vi "main-all-channels.vi"() -> ()   [LabVIEW 2024]
uses:
  controls/thermocouple-input-cluster.ctl
  controls/analog-input-cluster.ctl
  controls/analog-output-cluster.ctl
  controls/digitial-input-cluster.ctl
  controls/digital-output-cluster.ctl
  controls/adam-module-select-tab.ctl
  controls/adam-5000-serial-settings.ctl
  controls/adam-5000-cmd-response.ctl
  controls/state-enum.ctl
  controls/adam-5000-all-chassis-data.ctl
  controls/adam-5000-all-module-datas.ctl
  controls/adam-5000-chassis-cmd-ack.ctl
  controls/adam-5000-chassis-module-types.ctl
  controls/adam-5000-DO-user-input.ctl
  controls/adam-5000-AO-user-input.ctl
panel:
  out "cmd-response:7":T1
  out "status-indicator:7":cluster{"Sampling":bool, "Ack":bool}
  in  "Slot 7: Module Type":T2(ring)=enum."empty"
  out "slot: 7":T3
  in  "7:Digital Outputs":T4
  out "7:Digital Inputs":T5
  in  "7:Analog Outputs":T6
  out "7:Analog Inputs":T7
  out "7:Thermocouple Inputs (degC)":T8
  out "cmd-response:6":T1
  out "status-indicator:6":cluster{"Sampling":bool, "Ack":bool}
  in  "Slot 6: Module Type":T2(ring)=enum."empty"
  out "slot: 6":T3
  in  "6:Digital Outputs":T4
  out "6:Digital Inputs":T5
  in  "6:Analog Outputs":T6
  out "6:Analog Inputs":T7
  out "6:Thermocouple Inputs (degC)":T8
  out "cmd-response:5":T1
  out "status-indicator:5":cluster{"Sampling":bool, "Ack":bool}
  in  "Slot 5: Module Type":T2(ring)=enum."Analog Output"
  out "slot: 5":T3
  in  "5:Digital Outputs":T4
  out "5:Digital Inputs":T5
  in  "5:Analog Outputs":T6
  out "5:Analog Inputs":T7
  out "5:Thermocouple Inputs (degC)":T8
  out "cmd-response:4":T1
  out "status-indicator:4":cluster{"Sampling":bool, "Ack":bool}
  in  "Slot 4: Module Type":T2(ring)=enum."Power Relay"
  out "slot: 4":T3
  in  "4:Digital Outputs":T4
  out "4:Digital Inputs":T5
  in  "4:Analog Outputs":T6
  out "4:Analog Inputs":T7
  out "4:Thermocouple Inputs (degC)":T8
  out "cmd-response:3":T1
  out "status-indicator:3":cluster{"Sampling":bool, "Ack":bool}
  in  "Slot 3: Module Type":T2(ring)=enum."Thermocouple"
  out "slot: 3":T3
  in  "3:Digital Outputs":T4
  out "3:Digital Inputs":T5
  in  "3:Analog Outputs":T6
  out "3:Analog Inputs":T7
  out "3:Thermocouple Inputs (degC)":T8
  out "cmd-response:2":T1
  out "status-indicator:2":cluster{"Sampling":bool, "Ack":bool}
  in  "Slot 2: Module Type":T2(ring)=enum."Analog Input"
  out "slot: 2":T3
  in  "2:Digital Outputs":T4
  out "2:Digital Inputs":T5
  in  "2:Analog Outputs":T6
  out "2:Analog Inputs":T7
  out "2:Thermocouple Inputs (degC)":T8
  out "cmd-response:1":T1
  out "status-indicator:1":cluster{"Sampling":bool, "Ack":bool}
  in  "Slot 1: Module Type":T2(ring)=enum."Thermocouple"
  out "slot: 1":T3
  in  "1:Digital Outputs":T4
  out "1:Digital Inputs":T5
  in  "1:Analog Outputs":T6
  out "1:Analog Inputs":T7
  out "1:Thermocouple Inputs (degC)":T8
  out "cmd-response:0":T1
  out "status-indicator:0":cluster{"Sampling":bool, "Ack":bool}
  in  "Slot 0: Module Type":T2(ring)=enum."Analog Input"
  out "slot: 0":T3
  in  "0:Digital Outputs":T4
  out "0:Digital Inputs":T5
  in  "0:Analog Outputs:":T6
  out "0:Analog Inputs":T7
  out "0:Thermocouple Inputs (degC)":T8
  out "Current Slot":i32
  in  "Chassis Settings":T9={"VISA resource name"="COM8", "baud rate (19200)"=19200, "Chassis ID"=1}
  out "Loop Time (mS)":u32
  out "Loop Counter":i32
  out "Write Success":bool
  out "error IO":errorcluster
  out "error":errorcluster
  in  "exit":bool
  # "ADAM 5000 Controller"
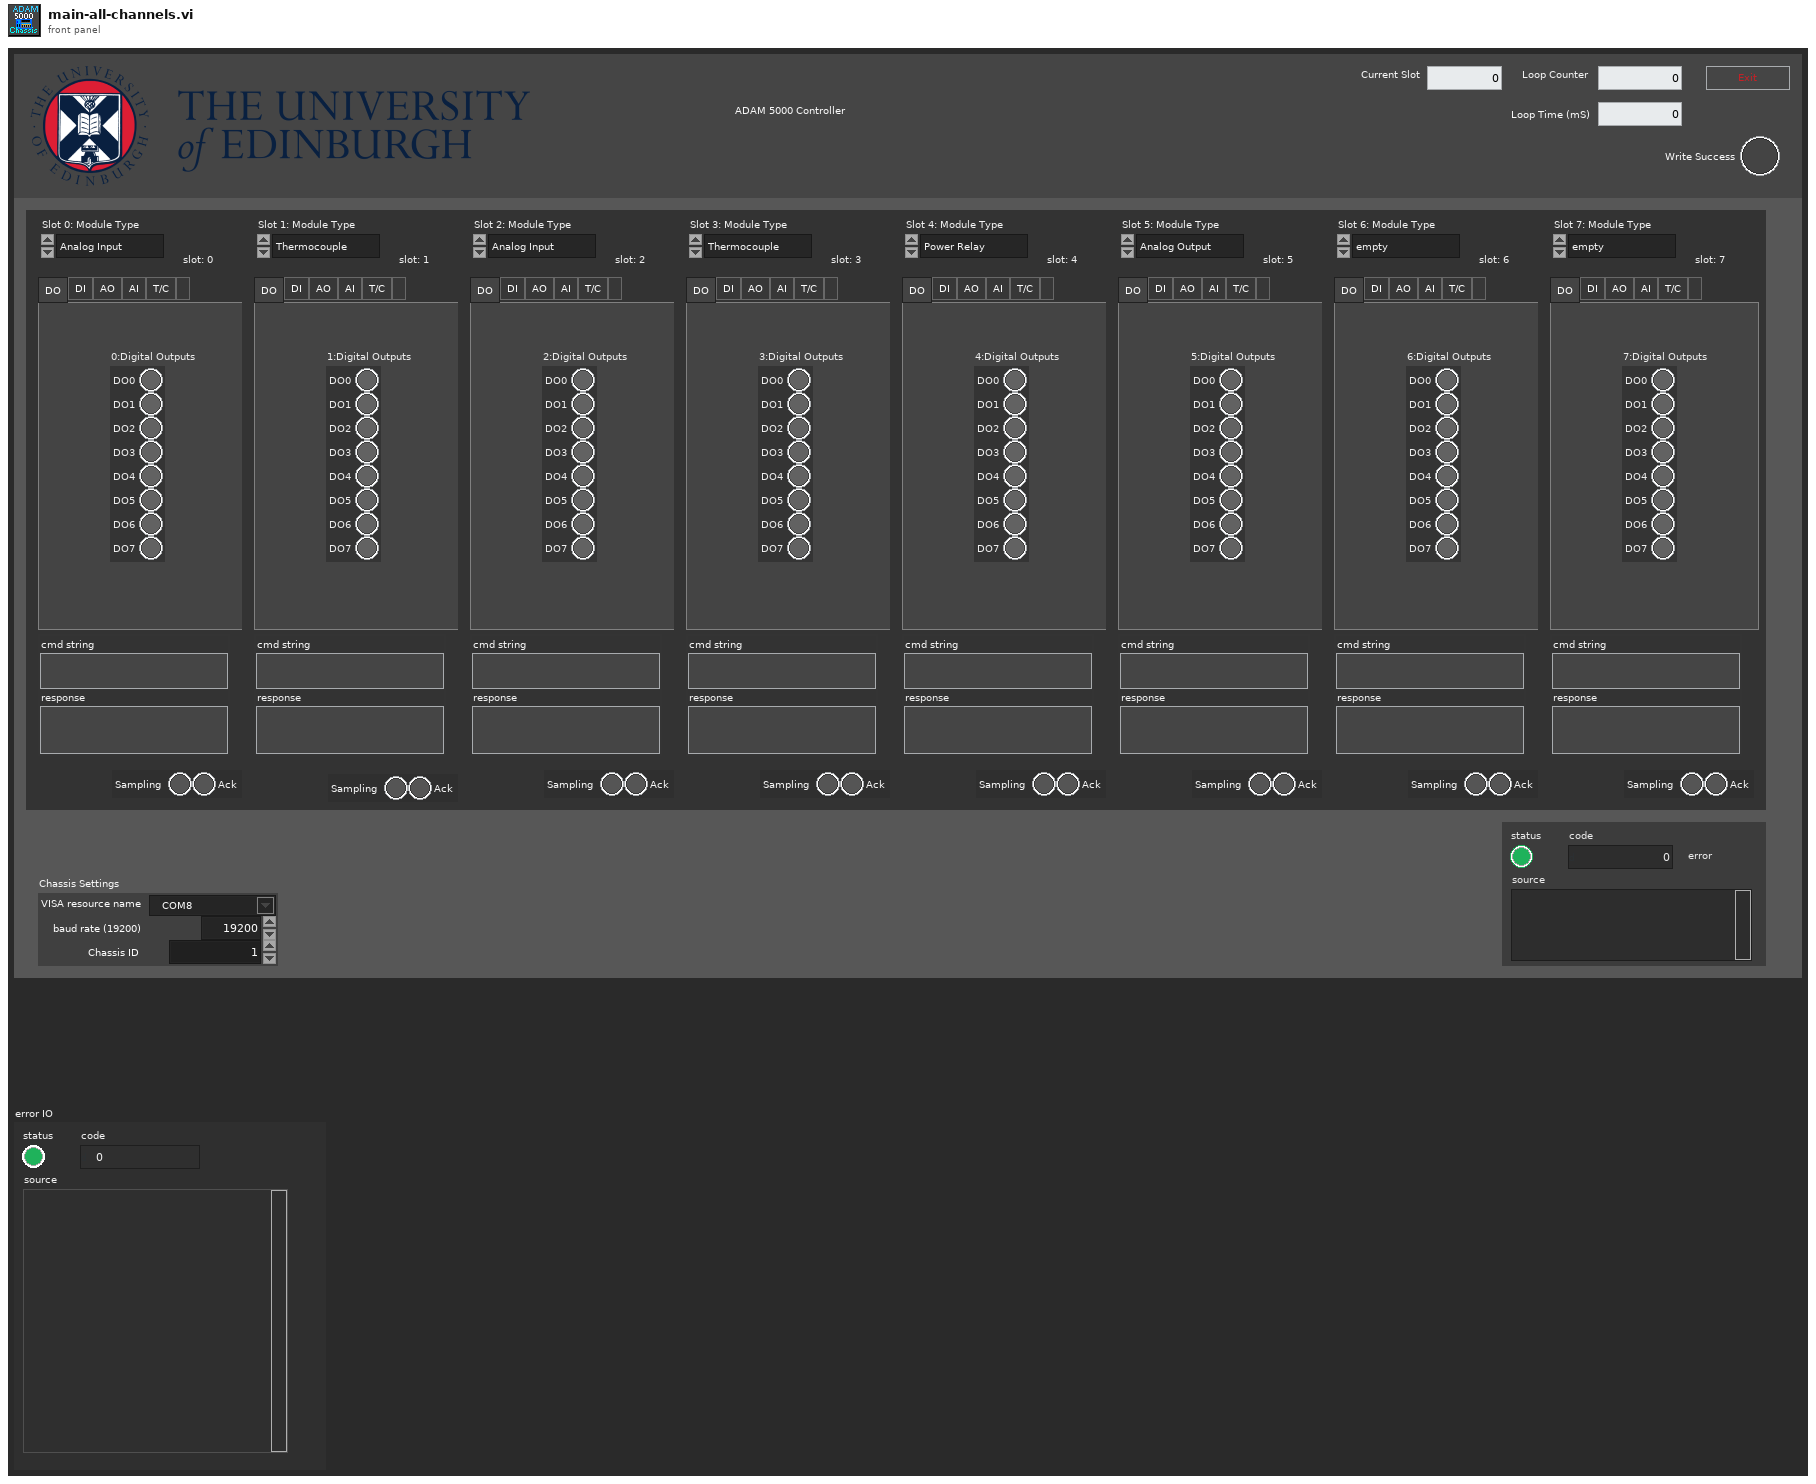
[diagram p1: front panel]
types:
  T1 = typedef "adam-5000-cmd-response.ctl" = cluster{"cmd string":string, "response":string}
  T2 = enum16{"Digital Output", "Digital Input", "Analog Output", "Analog Input", "Thermocouple", "Power Relay", "empty"}
  T3 = typedef "adam-module-select-tab.ctl" = enum32{"DO", "DI", "AO", "AI", "T/C", ""}
  T4 = typedef "digital-output-cluster.ctl" = cluster{"DO0":bool, "DO1":bool, "DO2":bool, "DO3":bool, "DO4":bool, "DO5":bool, "DO6":bool, "DO7":bool}
  T5 = typedef "digitial-input-cluster.ctl" = cluster{"DI0":bool, "DI1":bool, "DI2":bool, "DI3":bool, "DI4":bool, "DI5":bool, "DI6":bool, "DI7":bool}
  T6 = typedef "analog-output-cluster.ctl" = cluster{"AO0":dbl, "AO1":dbl, "AO2":dbl, "AO3":dbl}
  T7 = typedef "analog-input-cluster.ctl" = cluster{"AI0":dbl, "AI1":dbl, "AI2":dbl, "AI3":dbl, "AI4":dbl, "AI5":dbl, "AI6":dbl, "AI7":dbl}
  T8 = typedef "thermocouple-input-cluster.ctl" = cluster{"TC0":dbl, "TC1":dbl, "TC2":dbl, "TC3":dbl, "TC4":dbl, "TC5":dbl, "TC6":dbl}
  T9 = typedef "adam-5000-serial-settings.ctl" = cluster{"VISA resource name":refnum<visa-resource-name>, "baud rate (19200)":u32, "Chassis ID":u8}
  T10 = typedef "adam-5000-chassis-cmd-ack.ctl" = cluster{"cmd-response:0":T1, "cmd-response:1":T1, "cmd-response:2":T1, "cmd-response:3":T1, "cmd-response:4":T1, "cmd-response:5":T1, "cmd-response:6":T1, "cmd-response:7":T1}
  T11 = typedef "adam-5000-all-chassis-data.ctl" = cluster{"slot:0":T12, "slot:1":T12, "slot:2":T12, "slot:3":T12, "slot:4":T12, "slot:5":T12, "slot:6":T12, "slot:7":T12}
  T12 = typedef "adam-5000-all-module-datas.ctl" = cluster{"Digital Outputs":T4, "Digital Inputs":T5, "Analog Outputs":T6, "Analog Inputs":T7, "Thermocouple Inputs (degC)":T8}
  T13 = typedef "state-enum.ctl" = enum16{"init", "wait", "manual", "start", "run", "reset", "stop", "exit"}
  T14 = typedef "adam-5000-AO-user-input.ctl" = cluster{"0:Analog Outputs":T6, "1:Analog Outputs":T6, "2:Analog Outputs":T6, "3:Analog Outputs":T6, "4:Analog Outputs":T6, "5:Analog Outputs":T6, "6:Analog Outputs":T6, "7:Analog Outputs":T6}
  T15 = typedef "adam-5000-DO-user-input.ctl" = cluster{"0:Digital Outputs":T4, "1:Digital Outputs":T4, "2:Digital Outputs":T4, "3:Digital Outputs":T4, "4:Digital Outputs":T4, "5:Digital Outputs":T4, "6:Digital Outputs":T4, "7:Digital Outputs":T4}
  T16 = typedef "adam-5000-chassis-module-types.ctl" = cluster{"Slot 0: Module Type":enum16{"Digital Output", "Digital Input", "Analog Output", "Analog Input", "Thermocouple", "Power Relay", "empty"}, "Slot 1: Module Type":enum16{"Digital Output", "Digital Input", "Analog Output", "Analog Input", "Thermocouple", "Power Relay", "empty"}, "Slot 2: Module Type":enum16{"Digital Output", "Digital Input", "Analog Output", "Analog Input", "Thermocouple", "Power Relay", "empty"}, "Slot 3: Module Type":enum16{"Digital Output", "Digital Input", "Analog Output", "Analog Input", "Thermocouple", "Power Relay", "empty"}, "Slot 4: Module Type":enum16{"Digital Output", "Digital Input", "Analog Output", "Analog Input", "Thermocouple", "Power Relay", "empty"}, "Slot 5: Module Type":enum16{"Digital Output", "Digital Input", "Analog Output", "Analog Input", "Thermocouple", "Power Relay", "empty"}, "Slot 6: Module Type":enum16{"Digital Output", "Digital Input", "Analog Output", "Analog Input", "Thermocouple", "Power Relay", "empty"}, "Slot 7: Module Type":enum16{"Digital Output", "Digital Input", "Analog Output", "Analog Input", "Thermocouple", "Power Relay", "empty"}}
  T17 = cluster{"status-indicator:0":refnum<vi>, "status-indicator:1":refnum<vi>, "status-indicator:2":refnum<vi>, "status-indicator:3":refnum<vi>, "status-indicator:4":refnum<vi>, "status-indicator:5":refnum<vi>, "status-indicator:6":refnum<vi>, "status-indicator:7":refnum<vi>}
  T18 = enum16{"Digital Output", "Digital Input", "Analog Output", "Analog Input", "Thermocouple", "Power Relay", "empty"}[]
  T19 = cluster{"[0]":T3, "[1]":T3, "[2]":T3, "[3]":T3, "[4]":T3, "[5]":T3, "[6]":T3, "[7]":T3, "[8]":T3}
  T20 = cluster{"[0]":T12, "[1]":T12, "[2]":T12, "[3]":T12, "[4]":T12, "[5]":T12, "[6]":T12, "[7]":T12, "[8]":T12}
  T21 = cluster{"[0]":T1, "[1]":T1, "[2]":T1, "[3]":T1, "[4]":T1, "[5]":T1, "[6]":T1, "[7]":T1, "[8]":T1}
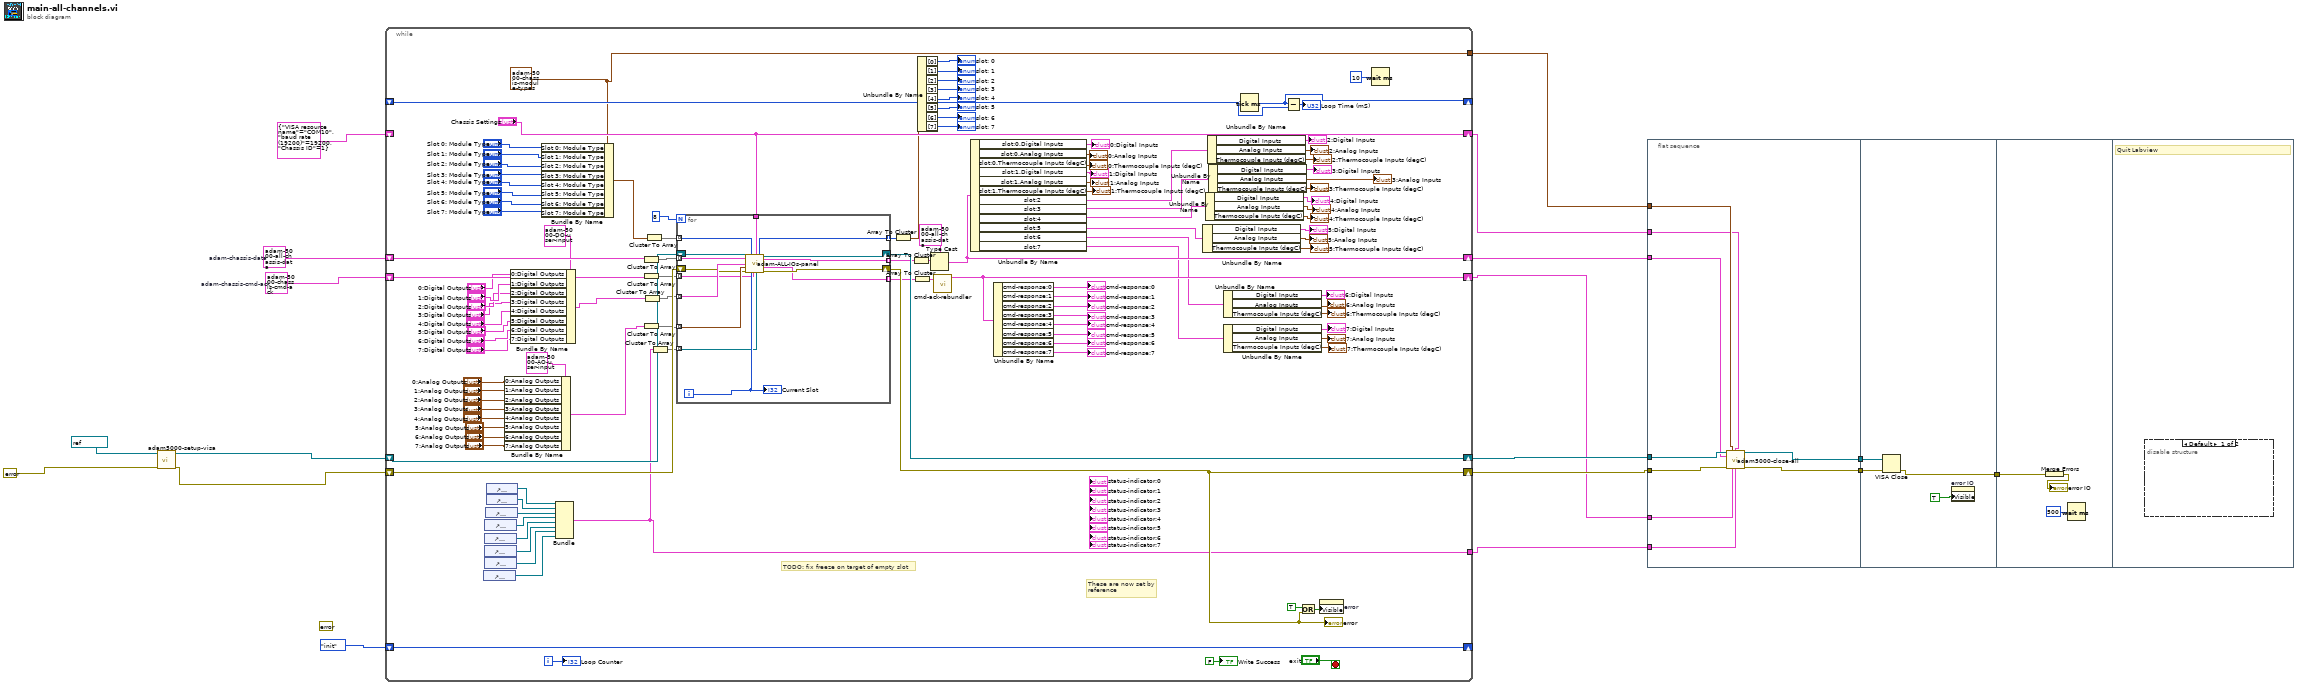
[diagram p0: block diagram]
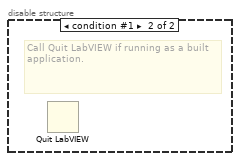
[diagram p2: hidden frame]
diagram:
  w10 = T10 {"cmd-response:0"={"cmd string"="", "response"=""}, "cmd-response:1"={"cmd string"="", "response"=""}, "cmd-response:2"={"cmd string"="", "response"=""}, "cmd-response:3"={"cmd string"="", "response"=""}, "cmd-response:4"={"cmd string"="", "response"=""}, "cmd-response:5"={"cmd string"="", "response"=""}, "cmd-response:6"={"cmd string"="", "response"=""}, "cmd-response:7"={"cmd string"="", "response"=""}}  # adam-chassis-cmd-ack
  w11 = T11 {"slot:0"={"Digital Outputs"={"DO0"=FALSE, "DO1"=FALSE, "DO2"=FALSE, "DO3"=FALSE, "DO4"=FALSE, "DO5"=FALSE, "DO6"=FALSE, "DO7"=FALSE}, "Digital Inputs"={"DI0"=FALSE, "DI1"=FALSE, "DI2"=FALSE, "DI3"=FALSE, "DI4"=FALSE, "DI5"=FALSE, "DI6"=FALSE, "DI7"=FALSE}, "Analog Outputs"={"AO0"=0.0, "AO1"=0.0, "AO2"=0.0, "AO3"=0.0}, "Analog Inputs"={"AI0"=0.0, "AI1"=0.0, "AI2"=0.0, "AI3"=0.0, "AI4"=0.0, "AI5"=0.0, "AI6"=0.0, "AI7"=0.0}, "Thermocouple Inputs (degC)"={"TC0"=0.0, "TC1"=0.0, "TC2"=0.0, "TC3"=0.0, "TC4"=0.0, "TC5"=0.0, "TC6"=0.0}}, "slot:1"={"Digital Outputs"={"DO0"=FALSE, "DO1"=FALSE, "DO2"=FALSE, "DO3"=FALSE, "DO4"=FALSE, "DO5"=FALSE, "DO6"=FALSE, "DO7"=FALSE}, "Digital Inputs"={"DI0"=FALSE, "DI1"=FALSE, "DI2"=FALSE, "DI3"=FALSE, "DI4"=FALSE, "DI5"=FALSE, "DI6"=FALSE, "DI7"=FALSE}, "Analog Outputs"={"AO0"=0.0, "AO1"=0.0, "AO2"=0.0, "AO3"=0.0}, "Analog Inputs"={"AI0"=0.0, "AI1"=0.0, "AI2"=0.0, "AI3"=0.0, "AI4"=0.0, "AI5"=0.0, "AI6"=0.0, "AI7"=0.0}, "Thermocouple Inputs (degC)"={"TC0"=0.0, "TC1"=0.0, "TC2"=0.0, "TC3"=0.0, "TC4"=0.0, "TC5"=0.0, "TC6"=0.0}}, "slot:2"={"Digital Outputs"={"DO0"=FALSE, "DO1"=FALSE, "DO2"=FALSE, "DO3"=FALSE, "DO4"=FALSE, "DO5"=FALSE, "DO6"=FALSE, "DO7"=FALSE}, "Digital Inputs"={"DI0"=FALSE, "DI1"=FALSE, "DI2"=FALSE, "DI3"=FALSE, "DI4"=FALSE, "DI5"=FALSE, "DI6"=FALSE, "DI7"=FALSE}, "Analog Outputs"={"AO0"=0.0, "AO1"=0.0, "AO2"=0.0, "AO3"=0.0}, "Analog Inputs"={"AI0"=0.0, "AI1"=0.0, "AI2"=0.0, "AI3"=0.0, "AI4"=0.0, "AI5"=0.0, "AI6"=0.0, "AI7"=0.0}, "Thermocouple Inputs (degC)"={"TC0"=0.0, "TC1"=0.0, "TC2"=0.0, "TC3"=0.0, "TC4"=0.0, "TC5"=0.0, "TC6"=0.0}}, "slot:3"={"Digital Outputs"={"DO0"=FALSE, "DO1"=FALSE, "DO2"=FALSE, "DO3"=FALSE, "DO4"=FALSE, "DO5"=FALSE, "DO6"=FALSE, "DO7"=FALSE}, "Digital Inputs"={"DI0"=FALSE, "DI1"=FALSE, "DI2"=FALSE, "DI3"=FALSE, "DI4"=FALSE, "DI5"=FALSE, "DI6"=FALSE, "DI7"=FALSE}, "Analog Outputs"={"AO0"=0.0, "AO1"=0.0, "AO2"=0.0, "AO3"=0.0}, "Analog Inputs"={"AI0"=0.0, "AI1"=0.0, "AI2"=0.0, "AI3"=0.0, "AI4"=0.0, "AI5"=0.0, "AI6"=0.0, "AI7"=0.0}, "Thermocouple Inputs (degC)"={"TC0"=0.0, "TC1"=0.0, "TC2"=0.0, "TC3"=0.0, "TC4"=0.0, "TC5"=0.0, "TC6"=0.0}}, "slot:4"={"Digital Outputs"={"DO0"=FALSE, "DO1"=FALSE, "DO2"=FALSE, "DO3"=FALSE, "DO4"=FALSE, "DO5"=FALSE, "DO6"=FALSE, "DO7"=FALSE}, "Digital Inputs"={"DI0"=FALSE, "DI1"=FALSE, "DI2"=FALSE, "DI3"=FALSE, "DI4"=FALSE, "DI5"=FALSE, "DI6"=FALSE, "DI7"=FALSE}, "Analog Outputs"={"AO0"=0.0, "AO1"=0.0, "AO2"=0.0, "AO3"=0.0}, "Analog Inputs"={"AI0"=0.0, "AI1"=0.0, "AI2"=0.0, "AI3"=0.0, "AI4"=0.0, "AI5"=0.0, "AI6"=0.0, "AI7"=0.0}, "Thermocouple Inputs (degC)"={"TC0"=0.0, "TC1"=0.0, "TC2"=0.0, "TC3"=0.0, "TC4"=0.0, "TC5"=0.0, "TC6"=0.0}}, "slot:5"={"Digital Outputs"={"DO0"=FALSE, "DO1"=FALSE, "DO2"=FALSE, "DO3"=FALSE, "DO4"=FALSE, "DO5"=FALSE, "DO6"=FALSE, "DO7"=FALSE}, "Digital Inputs"={"DI0"=FALSE, "DI1"=FALSE, "DI2"=FALSE, "DI3"=FALSE, "DI4"=FALSE, "DI5"=FALSE, "DI6"=FALSE, "DI7"=FALSE}, "Analog Outputs"={"AO0"=0.0, "AO1"=0.0, "AO2"=0.0, "AO3"=0.0}, "Analog Inputs"={"AI0"=0.0, "AI1"=0.0, "AI2"=0.0, "AI3"=0.0, "AI4"=0.0, "AI5"=0.0, "AI6"=0.0, "AI7"=0.0}, "Thermocouple Inputs (degC)"={"TC0"=0.0, "TC1"=0.0, "TC2"=0.0, "TC3"=0.0, "TC4"=0.0, "TC5"=0.0, "TC6"=0.0}}, "slot:6"={"Digital Outputs"={"DO0"=FALSE, "DO1"=FALSE, "DO2"=FALSE, "DO3"=FALSE, "DO4"=FALSE, "DO5"=FALSE, "DO6"=FALSE, "DO7"=FALSE}, "Digital Inputs"={"DI0"=FALSE, "DI1"=FALSE, "DI2"=FALSE, "DI3"=FALSE, "DI4"=FALSE, "DI5"=FALSE, "DI6"=FALSE, "DI7"=FALSE}, "Analog Outputs"={"AO0"=0.0, "AO1"=0.0, "AO2"=0.0, "AO3"=0.0}, "Analog Inputs"={"AI0"=0.0, "AI1"=0.0, "AI2"=0.0, "AI3"=0.0, "AI4"=0.0, "AI5"=0.0, "AI6"=0.0, "AI7"=0.0}, "Thermocouple Inputs (degC)"={"TC0"=0.0, "TC1"=0.0, "TC2"=0.0, "TC3"=0.0, "TC4"=0.0, "TC5"=0.0, "TC6"=0.0}}, "slot:7"={"Digital Outputs"={"DO0"=FALSE, "DO1"=FALSE, "DO2"=FALSE, "DO3"=FALSE, "DO4"=FALSE, "DO5"=FALSE, "DO6"=FALSE, "DO7"=FALSE}, "Digital Inputs"={"DI0"=FALSE, "DI1"=FALSE, "DI2"=FALSE, "DI3"=FALSE, "DI4"=FALSE, "DI5"=FALSE, "DI6"=FALSE, "DI7"=FALSE}, "Analog Outputs"={"AO0"=0.0, "AO1"=0.0, "AO2"=0.0, "AO3"=0.0}, "Analog Inputs"={"AI0"=0.0, "AI1"=0.0, "AI2"=0.0, "AI3"=0.0, "AI4"=0.0, "AI5"=0.0, "AI6"=0.0, "AI7"=0.0}, "Thermocouple Inputs (degC)"={"TC0"=0.0, "TC1"=0.0, "TC2"=0.0, "TC3"=0.0, "TC4"=0.0, "TC5"=0.0, "TC6"=0.0}}}  # adam-chassis-data
  (unwired) errorcluster {"status"=FALSE, "code"=0, "source"=""} ("error")
  n1 = call "adam5000-setup-visa.vi"("error in"=errorcluster {"status"=FALSE, "code"=0, "source"=""}, "VISA Refnum in"=refnum<visa-resource-name> "COM8") -> ("error out"=w8:errorcluster, "VISA Refnum out"=w7:refnum<visa-resource-name>)  [unwired: 8 in]
  n2 = while {
    shift-right: [w128] -> _
    shift-left: state-enum."init" ("state-enum") -> [w128]
    shift-right: [w104] -> w17
    shift-left: w8 -> [w116]
    shift-right: [w131] -> _
    shift-left: _ -> [w133]
    shift-right: ["Chassis Settings"] -> w2
    shift-left: T9 {"VISA resource name"="COM10", "baud rate (19200)"=19200, "Chassis ID"=1} ("Chassis Settings") -> [_]
    shift-right: [w115] -> w12
    shift-left: w7 -> [w117]
    shift-right: [w105] -> w5
    shift-left: w11 -> [w114]
    shift-right: [w90] -> w4
    shift-left: w10 -> [w112]
    tunnel: [w20] -> w3
    tunnel: [w19] -> w1
    i -> [w134]
    stop <- "exit" stop-if-true
    w20 = T16 {"Slot 0: Module Type"=enum."Digital Output", "Slot 1: Module Type"=enum."Digital Output", "Slot 2: Module Type"=enum."Digital Output", "Slot 3: Module Type"=enum."Digital Output", "Slot 4: Module Type"=enum."Digital Output", "Slot 5: Module Type"=enum."Digital Output", "Slot 6: Module Type"=enum."Digital Output", "Slot 7: Module Type"=enum."Digital Output"} ("cluster")
    # "TODO: fix freeze on target of empty slot"
    # "These are now set by\nreference"
    n3 = control-ref of="status-indicator:7"() -> (w50:refnum<vi>)
    n4 = control-ref of="status-indicator:4"() -> (w53:refnum<vi>)
    n5 = control-ref of="status-indicator:5"() -> (w52:refnum<vi>)
    n6 = control-ref of="status-indicator:3"() -> (w54:refnum<vi>)
    n7 = control-ref of="status-indicator:6"() -> (w51:refnum<vi>)
    n8 = control-ref of="status-indicator:2"() -> (w84:refnum<vi>)
    n9 = control-ref of="status-indicator:0"() -> (w101:refnum<vi>)
    n10 = control-ref of="status-indicator:1"() -> (w100:refnum<vi>)
    n11 = Bundle By Name(cluster=T14 {"0:Analog Outputs"={"AO0"=0.0, "AO1"=0.0, "AO2"=0.0, "AO3"=0.0}, "1:Analog Outputs"={"AO0"=0.0, "AO1"=0.0, "AO2"=0.0, "AO3"=0.0}, "2:Analog Outputs"={"AO0"=0.0, "AO1"=0.0, "AO2"=0.0, "AO3"=0.0}, "3:Analog Outputs"={"AO0"=0.0, "AO1"=0.0, "AO2"=0.0, "AO3"=0.0}, "4:Analog Outputs"={"AO0"=0.0, "AO1"=0.0, "AO2"=0.0, "AO3"=0.0}, "5:Analog Outputs"={"AO0"=0.0, "AO1"=0.0, "AO2"=0.0, "AO3"=0.0}, "6:Analog Outputs"={"AO0"=0.0, "AO1"=0.0, "AO2"=0.0, "AO3"=0.0}, "7:Analog Outputs"={"AO0"=0.0, "AO1"=0.0, "AO2"=0.0, "AO3"=0.0}}, "0:Analog Outputs"="0:Analog Outputs:", "1:Analog Outputs"="1:Analog Outputs", "2:Analog Outputs"="2:Analog Outputs", "3:Analog Outputs"="3:Analog Outputs", "4:Analog Outputs"="4:Analog Outputs", "5:Analog Outputs"="5:Analog Outputs", "6:Analog Outputs"="6:Analog Outputs", "7:Analog Outputs"="7:Analog Outputs") -> (w29:T14)
    n12 = Bundle By Name(cluster=T15 {"0:Digital Outputs"={"DO0"=FALSE, "DO1"=FALSE, "DO2"=FALSE, "DO3"=FALSE, "DO4"=FALSE, "DO5"=FALSE, "DO6"=FALSE, "DO7"=FALSE}, "1:Digital Outputs"={"DO0"=FALSE, "DO1"=FALSE, "DO2"=FALSE, "DO3"=FALSE, "DO4"=FALSE, "DO5"=FALSE, "DO6"=FALSE, "DO7"=FALSE}, "2:Digital Outputs"={"DO0"=FALSE, "DO1"=FALSE, "DO2"=FALSE, "DO3"=FALSE, "DO4"=FALSE, "DO5"=FALSE, "DO6"=FALSE, "DO7"=FALSE}, "3:Digital Outputs"={"DO0"=FALSE, "DO1"=FALSE, "DO2"=FALSE, "DO3"=FALSE, "DO4"=FALSE, "DO5"=FALSE, "DO6"=FALSE, "DO7"=FALSE}, "4:Digital Outputs"={"DO0"=FALSE, "DO1"=FALSE, "DO2"=FALSE, "DO3"=FALSE, "DO4"=FALSE, "DO5"=FALSE, "DO6"=FALSE, "DO7"=FALSE}, "5:Digital Outputs"={"DO0"=FALSE, "DO1"=FALSE, "DO2"=FALSE, "DO3"=FALSE, "DO4"=FALSE, "DO5"=FALSE, "DO6"=FALSE, "DO7"=FALSE}, "6:Digital Outputs"={"DO0"=FALSE, "DO1"=FALSE, "DO2"=FALSE, "DO3"=FALSE, "DO4"=FALSE, "DO5"=FALSE, "DO6"=FALSE, "DO7"=FALSE}, "7:Digital Outputs"={"DO0"=FALSE, "DO1"=FALSE, "DO2"=FALSE, "DO3"=FALSE, "DO4"=FALSE, "DO5"=FALSE, "DO6"=FALSE, "DO7"=FALSE}}, "0:Digital Outputs"="0:Digital Outputs", "1:Digital Outputs"="1:Digital Outputs", "2:Digital Outputs"="2:Digital Outputs", "3:Digital Outputs"="3:Digital Outputs", "4:Digital Outputs"="4:Digital Outputs", "5:Digital Outputs"="5:Digital Outputs", "6:Digital Outputs"="6:Digital Outputs", "7:Digital Outputs"="7:Digital Outputs") -> (w39:T15)
    n13 = Bundle By Name(cluster=w20, "Slot 0: Module Type"="Slot 0: Module Type", "Slot 1: Module Type"="Slot 1: Module Type", "Slot 2: Module Type"="Slot 2: Module Type", "Slot 3: Module Type"="Slot 3: Module Type", "Slot 4: Module Type"="Slot 4: Module Type", "Slot 5: Module Type"="Slot 5: Module Type", "Slot 6: Module Type"="Slot 6: Module Type", "Slot 7: Module Type"="Slot 7: Module Type") -> (w41:T16)
    n14 = Bundle("status-indicator:0"=w101, "status-indicator:1"=w100, "status-indicator:2"=w84, "status-indicator:3"=w54, "status-indicator:4"=w53, "status-indicator:5"=w52, "status-indicator:6"=w51, "status-indicator:7"=w50) -> (w19:T17)  [unwired: 1 in]
    n15 = Cluster To Array(cluster=w112) -> (array=w111:T1[])
    n16 = Cluster To Array(cluster=w114) -> (array=w113:T12[])
    n17 = Cluster To Array(cluster=w29) -> (array=w109:T6[])
    n18 = Cluster To Array(cluster=w39) -> (array=w110:T4[])
    n19 = Cluster To Array(cluster=w41) -> (array=w103:T18)
    n20 = Cluster To Array(cluster=w19) -> (array=w99:refnum<vi>[])
    n21 = for {
      N: 8 -> [_]
      shift-right: [w142] -> w104
      shift-left: w116 -> [w143]
      shift-right: [w148] -> w115
      shift-left: w117 -> [w147]
      tunnel: w113 -> [w146] mode=indexing
      tunnel: w111 -> [w138] mode=indexing
      tunnel: w110 -> [w145] mode=indexing
      tunnel: w109 -> [w144] mode=indexing
      tunnel: "Chassis Settings" -> [w150]
      tunnel: w103 -> [w151] mode=indexing
      tunnel: w99 -> [w137] mode=indexing
      tunnel: [w149] -> w98 mode=indexing
      tunnel: [w141] -> w97 mode=indexing
      tunnel: [w140] -> w96 mode=indexing
      i -> [w139]
      n22 = call "adam-ALL-IOs-panel.vi"("VISA Refnum in"=w147, "ADAM-5000-data-current"=w146, "Digital Outputs"=w145, "Analog Outputs"=w144, "error in (no error)"=w143, "Module Type"=w151, "chassis-slot"=w139, "cmd-response in"=w138, "Chassis Settings"=w150, "reference"=w137) -> ("slot: x"=w149:T3, "VISA Refnum out"=w148:refnum<visa-resource-name>, "ADAM-5000-data-new"=w141:T12, "cmd-response out"=w140:T1, "error out"=w142:errorcluster)  [unwired: 5 in]
      "Current Slot" <- w139
    }
    "error" <- w104
    n23 = Array To Cluster(array=w98) -> (cluster=w102:T19)
    n24 = Array To Cluster(array=w97) -> (cluster=w107:T20)
    n25 = Array To Cluster(array=w96) -> (cluster=w89:T21)
    n26 = Unbundle By Name(w102) -> ("[0]"=→"slot: 0":T3, "[1]"=→"slot: 1":T3, "[2]"=→"slot: 2":T3, "[3]"=→"slot: 3":T3, "[4]"=→"slot: 4":T3, "[5]"=→"slot: 5":T3, "[6]"=→"slot: 6":T3, "[7]"=→"slot: 7":T3)
    n27 = Type Cast(type=T11 {"slot:0"={"Digital Outputs"={"DO0"=FALSE, "DO1"=FALSE, "DO2"=FALSE, "DO3"=FALSE, "DO4"=FALSE, "DO5"=FALSE, "DO6"=FALSE, "DO7"=FALSE}, "Digital Inputs"={"DI0"=FALSE, "DI1"=FALSE, "DI2"=FALSE, "DI3"=FALSE, "DI4"=FALSE, "DI5"=FALSE, "DI6"=FALSE, "DI7"=FALSE}, "Analog Outputs"={"AO0"=0.0, "AO1"=0.0, "AO2"=0.0, "AO3"=0.0}, "Analog Inputs"={"AI0"=0.0, "AI1"=0.0, "AI2"=0.0, "AI3"=0.0, "AI4"=0.0, "AI5"=0.0, "AI6"=0.0, "AI7"=0.0}, "Thermocouple Inputs (degC)"={"TC0"=0.0, "TC1"=0.0, "TC2"=0.0, "TC3"=0.0, "TC4"=0.0, "TC5"=0.0, "TC6"=0.0}}, "slot:1"={"Digital Outputs"={"DO0"=FALSE, "DO1"=FALSE, "DO2"=FALSE, "DO3"=FALSE, "DO4"=FALSE, "DO5"=FALSE, "DO6"=FALSE, "DO7"=FALSE}, "Digital Inputs"={"DI0"=FALSE, "DI1"=FALSE, "DI2"=FALSE, "DI3"=FALSE, "DI4"=FALSE, "DI5"=FALSE, "DI6"=FALSE, "DI7"=FALSE}, "Analog Outputs"={"AO0"=0.0, "AO1"=0.0, "AO2"=0.0, "AO3"=0.0}, "Analog Inputs"={"AI0"=0.0, "AI1"=0.0, "AI2"=0.0, "AI3"=0.0, "AI4"=0.0, "AI5"=0.0, "AI6"=0.0, "AI7"=0.0}, "Thermocouple Inputs (degC)"={"TC0"=0.0, "TC1"=0.0, "TC2"=0.0, "TC3"=0.0, "TC4"=0.0, "TC5"=0.0, "TC6"=0.0}}, "slot:2"={"Digital Outputs"={"DO0"=FALSE, "DO1"=FALSE, "DO2"=FALSE, "DO3"=FALSE, "DO4"=FALSE, "DO5"=FALSE, "DO6"=FALSE, "DO7"=FALSE}, "Digital Inputs"={"DI0"=FALSE, "DI1"=FALSE, "DI2"=FALSE, "DI3"=FALSE, "DI4"=FALSE, "DI5"=FALSE, "DI6"=FALSE, "DI7"=FALSE}, "Analog Outputs"={"AO0"=0.0, "AO1"=0.0, "AO2"=0.0, "AO3"=0.0}, "Analog Inputs"={"AI0"=0.0, "AI1"=0.0, "AI2"=0.0, "AI3"=0.0, "AI4"=0.0, "AI5"=0.0, "AI6"=0.0, "AI7"=0.0}, "Thermocouple Inputs (degC)"={"TC0"=0.0, "TC1"=0.0, "TC2"=0.0, "TC3"=0.0, "TC4"=0.0, "TC5"=0.0, "TC6"=0.0}}, "slot:3"={"Digital Outputs"={"DO0"=FALSE, "DO1"=FALSE, "DO2"=FALSE, "DO3"=FALSE, "DO4"=FALSE, "DO5"=FALSE, "DO6"=FALSE, "DO7"=FALSE}, "Digital Inputs"={"DI0"=FALSE, "DI1"=FALSE, "DI2"=FALSE, "DI3"=FALSE, "DI4"=FALSE, "DI5"=FALSE, "DI6"=FALSE, "DI7"=FALSE}, "Analog Outputs"={"AO0"=0.0, "AO1"=0.0, "AO2"=0.0, "AO3"=0.0}, "Analog Inputs"={"AI0"=0.0, "AI1"=0.0, "AI2"=0.0, "AI3"=0.0, "AI4"=0.0, "AI5"=0.0, "AI6"=0.0, "AI7"=0.0}, "Thermocouple Inputs (degC)"={"TC0"=0.0, "TC1"=0.0, "TC2"=0.0, "TC3"=0.0, "TC4"=0.0, "TC5"=0.0, "TC6"=0.0}}, "slot:4"={"Digital Outputs"={"DO0"=FALSE, "DO1"=FALSE, "DO2"=FALSE, "DO3"=FALSE, "DO4"=FALSE, "DO5"=FALSE, "DO6"=FALSE, "DO7"=FALSE}, "Digital Inputs"={"DI0"=FALSE, "DI1"=FALSE, "DI2"=FALSE, "DI3"=FALSE, "DI4"=FALSE, "DI5"=FALSE, "DI6"=FALSE, "DI7"=FALSE}, "Analog Outputs"={"AO0"=0.0, "AO1"=0.0, "AO2"=0.0, "AO3"=0.0}, "Analog Inputs"={"AI0"=0.0, "AI1"=0.0, "AI2"=0.0, "AI3"=0.0, "AI4"=0.0, "AI5"=0.0, "AI6"=0.0, "AI7"=0.0}, "Thermocouple Inputs (degC)"={"TC0"=0.0, "TC1"=0.0, "TC2"=0.0, "TC3"=0.0, "TC4"=0.0, "TC5"=0.0, "TC6"=0.0}}, "slot:5"={"Digital Outputs"={"DO0"=FALSE, "DO1"=FALSE, "DO2"=FALSE, "DO3"=FALSE, "DO4"=FALSE, "DO5"=FALSE, "DO6"=FALSE, "DO7"=FALSE}, "Digital Inputs"={"DI0"=FALSE, "DI1"=FALSE, "DI2"=FALSE, "DI3"=FALSE, "DI4"=FALSE, "DI5"=FALSE, "DI6"=FALSE, "DI7"=FALSE}, "Analog Outputs"={"AO0"=0.0, "AO1"=0.0, "AO2"=0.0, "AO3"=0.0}, "Analog Inputs"={"AI0"=0.0, "AI1"=0.0, "AI2"=0.0, "AI3"=0.0, "AI4"=0.0, "AI5"=0.0, "AI6"=0.0, "AI7"=0.0}, "Thermocouple Inputs (degC)"={"TC0"=0.0, "TC1"=0.0, "TC2"=0.0, "TC3"=0.0, "TC4"=0.0, "TC5"=0.0, "TC6"=0.0}}, "slot:6"={"Digital Outputs"={"DO0"=FALSE, "DO1"=FALSE, "DO2"=FALSE, "DO3"=FALSE, "DO4"=FALSE, "DO5"=FALSE, "DO6"=FALSE, "DO7"=FALSE}, "Digital Inputs"={"DI0"=FALSE, "DI1"=FALSE, "DI2"=FALSE, "DI3"=FALSE, "DI4"=FALSE, "DI5"=FALSE, "DI6"=FALSE, "DI7"=FALSE}, "Analog Outputs"={"AO0"=0.0, "AO1"=0.0, "AO2"=0.0, "AO3"=0.0}, "Analog Inputs"={"AI0"=0.0, "AI1"=0.0, "AI2"=0.0, "AI3"=0.0, "AI4"=0.0, "AI5"=0.0, "AI6"=0.0, "AI7"=0.0}, "Thermocouple Inputs (degC)"={"TC0"=0.0, "TC1"=0.0, "TC2"=0.0, "TC3"=0.0, "TC4"=0.0, "TC5"=0.0, "TC6"=0.0}}, "slot:7"={"Digital Outputs"={"DO0"=FALSE, "DO1"=FALSE, "DO2"=FALSE, "DO3"=FALSE, "DO4"=FALSE, "DO5"=FALSE, "DO6"=FALSE, "DO7"=FALSE}, "Digital Inputs"={"DI0"=FALSE, "DI1"=FALSE, "DI2"=FALSE, "DI3"=FALSE, "DI4"=FALSE, "DI5"=FALSE, "DI6"=FALSE, "DI7"=FALSE}, "Analog Outputs"={"AO0"=0.0, "AO1"=0.0, "AO2"=0.0, "AO3"=0.0}, "Analog Inputs"={"AI0"=0.0, "AI1"=0.0, "AI2"=0.0, "AI3"=0.0, "AI4"=0.0, "AI5"=0.0, "AI6"=0.0, "AI7"=0.0}, "Thermocouple Inputs (degC)"={"TC0"=0.0, "TC1"=0.0, "TC2"=0.0, "TC3"=0.0, "TC4"=0.0, "TC5"=0.0, "TC6"=0.0}}}, x=w107) -> (*(type *) &x=w105:T11)
    n28 = call "cmd-ack-rebundler.vi"("cmd-response-in"=w89) -> ("adam-chassis-cmd-response-out"=w90:T10)  [unwired: 10 in]
    n29 = Unbundle By Name(w105) -> ("slot:0.Digital Inputs"=→"0:Digital Inputs":T5, "slot:0.Analog Inputs"=→"0:Analog Inputs":T7, "slot:0.Thermocouple Inputs (degC)"=→"0:Thermocouple Inputs (degC)":T8, "slot:1.Digital Inputs"=→"1:Digital Inputs":T5, "slot:1.Analog Inputs"=→"1:Analog Inputs":T7, "slot:1.Thermocouple Inputs (degC)"=→"1:Thermocouple Inputs (degC)":T8, "slot:2"=w94:T12, "slot:3"=w85:T12, "slot:4"=w79:T12, "slot:5"=w66:T12, "slot:6"=w62:T12, "slot:7"=w61:T12)
    n30 = Unbundle By Name(w90) -> ("cmd-response:0"=→"cmd-response:0":T1, "cmd-response:1"=→"cmd-response:1":T1, "cmd-response:2"=→"cmd-response:2":T1, "cmd-response:3"=→"cmd-response:3":T1, "cmd-response:4"=→"cmd-response:4":T1, "cmd-response:5"=→"cmd-response:5":T1, "cmd-response:6"=→"cmd-response:6":T1, "cmd-response:7"=→"cmd-response:7":T1)
    n31 = Unbundle By Name(w66) -> ("Digital Inputs"=→"5:Digital Inputs":T5, "Analog Inputs"=→"5:Analog Inputs":T7, "Thermocouple Inputs (degC)"=→"5:Thermocouple Inputs (degC)":T8)
    n32 = Unbundle By Name(w79) -> ("Digital Inputs"=→"4:Digital Inputs":T5, "Analog Inputs"=→"4:Analog Inputs":T7, "Thermocouple Inputs (degC)"=→"4:Thermocouple Inputs (degC)":T8)
    n33 = Unbundle By Name(w94) -> ("Digital Inputs"=→"2:Digital Inputs":T5, "Analog Inputs"=→"2:Analog Inputs":T7, "Thermocouple Inputs (degC)"=→"2:Thermocouple Inputs (degC)":T8)
    n34 = Unbundle By Name(w85) -> ("Digital Inputs"=→"3:Digital Inputs":T5, "Analog Inputs"=→"3:Analog Inputs":T7, "Thermocouple Inputs (degC)"=→"3:Thermocouple Inputs (degC)":T8)
    n35 = Unbundle By Name(w62) -> ("Digital Inputs"=→"6:Digital Inputs":T5, "Analog Inputs"=→"6:Analog Inputs":T7, "Thermocouple Inputs (degC)"=→"6:Thermocouple Inputs (degC)":T8)
    n36 = Unbundle By Name(w61) -> ("Digital Inputs"=→"7:Digital Inputs":T5, "Analog Inputs"=→"7:Analog Inputs":T7, "Thermocouple Inputs (degC)"=→"7:Thermocouple Inputs (degC)":T8)
    n37 = Tick Count (ms)() -> (millisecond timer value=w131:u32)
    n38 = Subtract(x=w131, y=w133) -> (x-y=→"Loop Time (mS)":u32)
    n39 = Or(x=TRUE ("Debug Mode"), y=w104) -> (x .or. y?=w130:bool)
    n40 = property on="error" class="Clust (strict)"("Visible"=w130) -> ()  [unwired: 2 in, 2 out]
    n41 = Wait (ms)(milliseconds to wait=u32 10) -> ()  [unwired: 1 out]
    "Write Success" <- FALSE ("Write Success")
    "Loop Counter" <- w134
  }
  n42 = flat-sequence {
    tunnel: w17 -> [w159]
    tunnel: [w157] -> w15
    tunnel: [w158] -> w14
    tunnel: w12 -> [w160]
    tunnel: w5 -> [w156]
    tunnel: w4 -> [w155]
    tunnel: w3 -> [w154]
    tunnel: w2 -> [w153]
    tunnel: w1 -> [w152]
    tunnel: [w161] -> w16
    tunnel: w15 -> [w162]
    tunnel: w14 -> [w163]
    tunnel: w16 -> [w165]
    frame #0 {
      n43 = call "adam5000-close-all.vi"("VISA Refnum in"=w160, "adam5000:module-type-select"=w154, "Chassis Settings in"=w153, "adam5000:all-data-in"=w156, "error in (no error)"=w159, "adam-chassis-cmd-ack"=w155, "adam5000:status-ref"=w152) -> ("VISA Refnum out"=w157:refnum<visa-resource-name>, "error out"=w158:errorcluster)  [unwired: 5 in, 2 out]
    }
    frame #1 {
      n44 = VISA Close(VISA resource name=w162, error in (no error)=w163) -> (error out=w161:errorcluster)
      n45 = property on="error IO" class="Clust (strict)"("Visible"=TRUE) -> ()  [unwired: 2 in, 2 out]
    }
    frame #2 {
      n46 = Merge Errors(w165) -> (→"error IO":errorcluster)
      n47 = Wait (ms)(milliseconds to wait=u32 500) -> ()  [unwired: 1 out]
    }
    frame #3 {
      # "Quit Labview"
      n48 = disable-structure "Conditional Disable Structure" shown="Default" {
        frame condition #0 (active) {
        }
        frame condition #1 {
          # "Call Quit LabVIEW if running as a built application."
          n49 = Quit LabVIEW() -> ()  [unwired: 1 in]
        }
      }
    }
  }
